vi "Write All History File.vi"(8 "error in (no error)":errorcluster, 10 "All History File":path, 11 "Data Manager in":refnum<class "Data Manager.lvclass">) -> (0 "error out":errorcluster, 3 "Data Manager out":refnum<class "Data Manager.lvclass">)   [LabVIEW 2020, in "Data Manager.lvclass"]
uses:
  Data Manager.lvclass
  Data Manager.lvclass/Data Manager.ctl
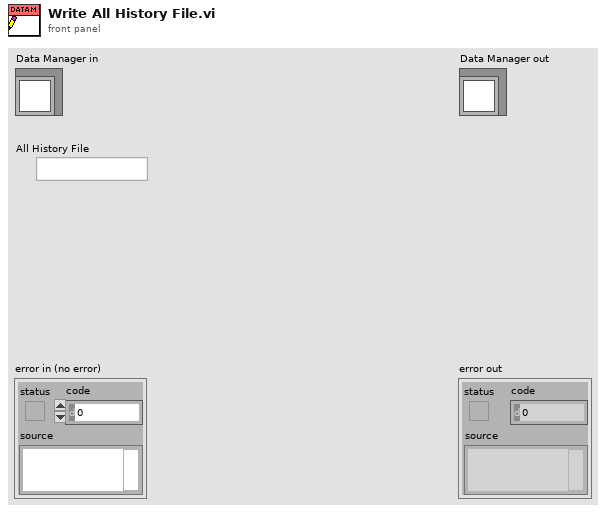
[diagram p1: front panel]
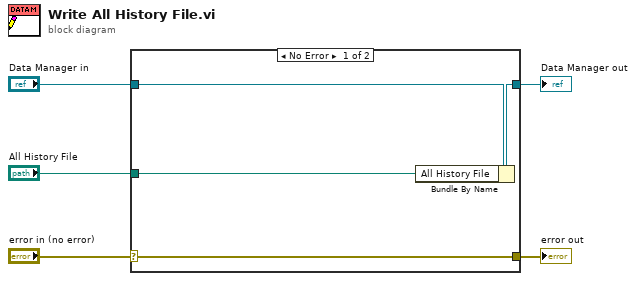
[diagram p0: block diagram]
diagram:
  n1 = case shown="No Error" "error in (no error)" {
    selector: "error in (no error)" -> [w9 w10]
    tunnel: [w9 w10] -> w4
    tunnel: [w7 w11] -> w2
    tunnel: "Data Manager in" -> [w8 w11]
    tunnel: "All History File" -> [w6 _]
    frame No Error {
      n2 = Bundle By Name(cluster=w8, "All History File"=w6) -> (w7:refnum<class "Data Manager.lvclass">)
    }
    frame Error {
    }
  }
  "error out" <- w4
  "Data Manager out" <- w2
